vi "get current and reset position.vi"(0 "VISA Refnum in":refnum<visa-resource-name>, 2 "DELAY (ms) in":u32, 3 "Dup Controller # in":string, 5 "error in (no error)":errorcluster) -> (10 "Dup Controller #":string, 11 "Reset displacement":ext, 14 "VISA Refnum out":refnum<visa-resource-name>, 15 "Delay (ms) out":u32, 16 "Response":string, 17 "Current position":i32, 19 "error out":errorcluster)   [LabVIEW 2014]
doc: "This vi is used to get the current position of the motor and the reset displacement value which has to be fed to reset"
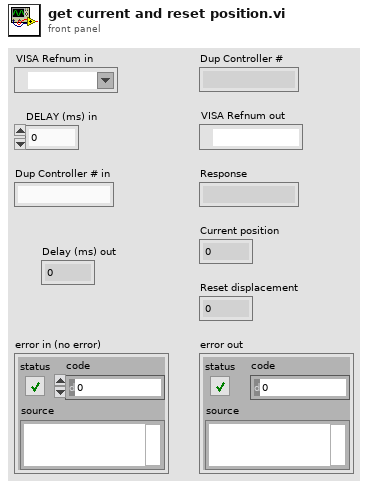
[diagram p1: front panel]
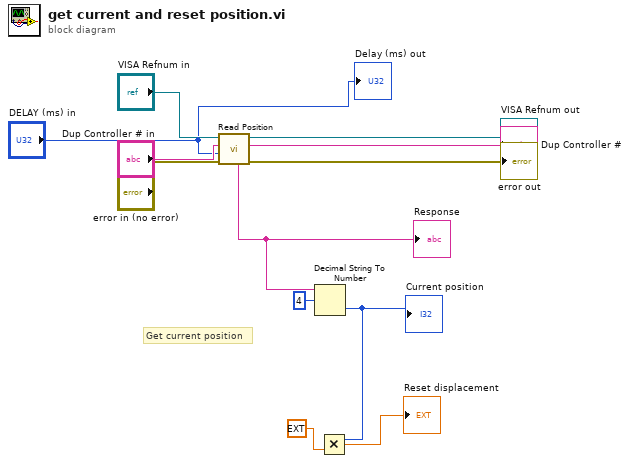
[diagram p0: block diagram]
diagram:
  # "Get current position"
  n1 = call <userlib>:"Read Position.vi"("error in (no error)"="error in (no error)", "Delay (ms)"="DELAY (ms) in", "Controller #"="Dup Controller # in", "VISA Handle"="VISA Refnum in") -> ("error out"=→"error out":errorcluster, "Response"=w3:string, "Dup Controller #"=→"Dup Controller #":string, "Dup VISA Handle"=→"VISA Refnum out":refnum<visa-resource-name>)  [unwired: 2 out]
  "Response" <- w3
  n2 = Decimal String To Number(string=w3, offset=4) -> (number=w8:i32)  [unwired: 2 out]
  "Current position" <- w8
  n3 = Multiply(x=w8, y=ext -1.0) -> (x*y=→"Reset displacement":ext)
  "Delay (ms) out" <- "DELAY (ms) in"
